vi "Stack_holderwise_total_bd_count_&_duration_Monthwise.vi"(0 "Refnum in":T1, 1 "BREAKDOWN_STK_HOLD_ID":i32=1, 2 "condition":string="Where BREAKDOWN_DATE between '%s'and '%s' and BREAKDOWN_STK_HOLD_ID ='%d'  ", 5 "Shift":string, 11 "error in (no error)":errorcluster) -> (4 "Refnum out":T1, 6 "Count out":string[](array[string]), 10 "appended array":dbl[](array[numeric]), 15 "error out":errorcluster)   [LabVIEW 2017]
uses:
  <vilib>/addons/database/Connection.llb/Conn ObjectReference.ctl
  <vilib>/addons/database/NI_Database_API.lvlib
panel:
  out "Table":string[][](array[string])
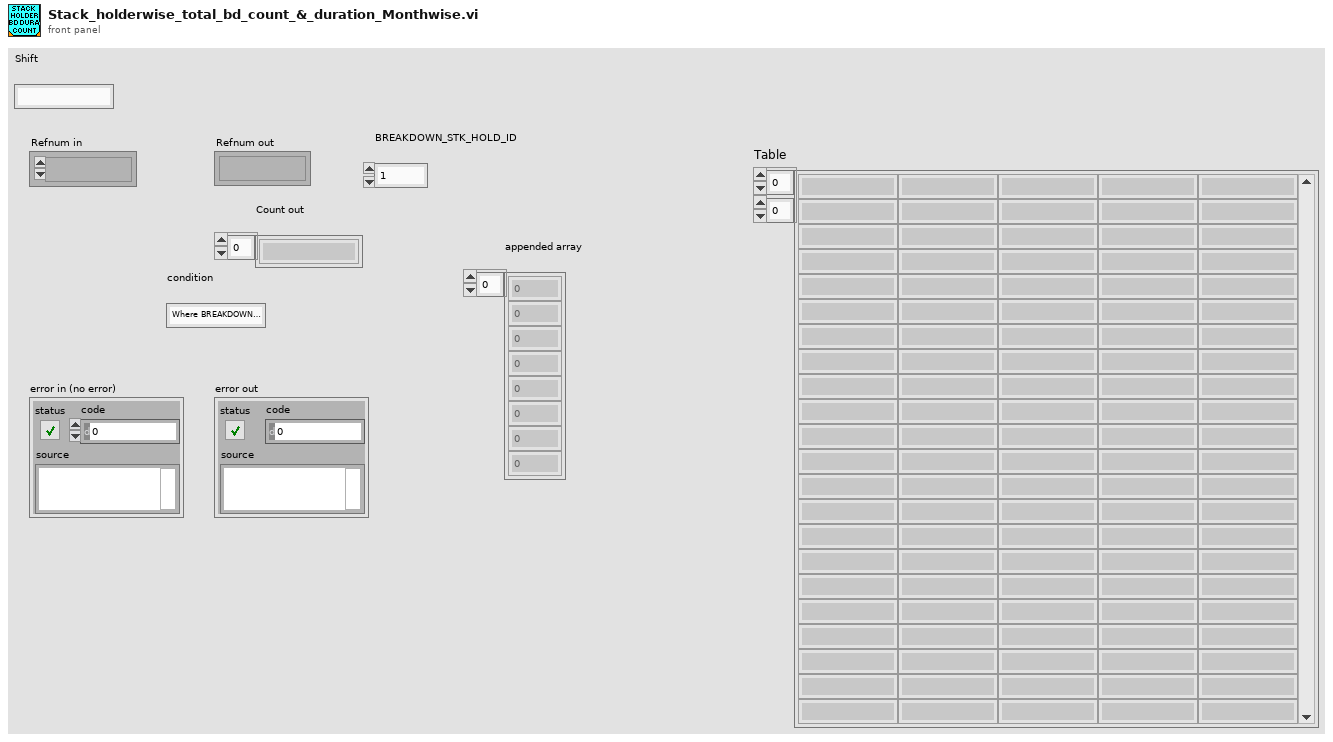
[diagram p1: front panel]
types:
  T1 = typedef "NI_Database_API.lvlib/Conn ObjectReference.ctl" = refnum<k1>
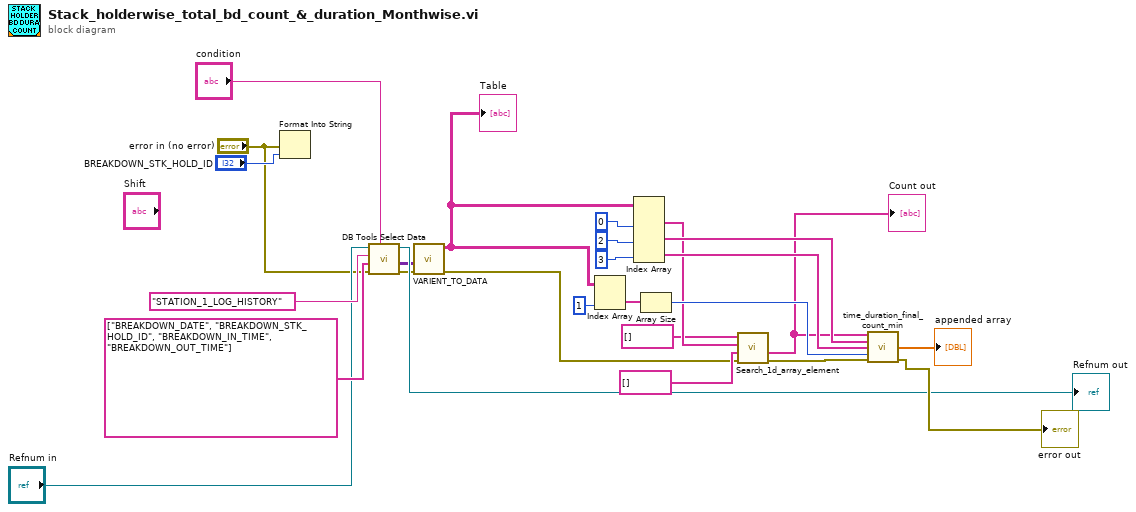
[diagram p0: block diagram]
diagram:
  n1 = Format Into String(error in="error in (no error)", "BREAKDOWN_STK_HOLD_ID") -> ()  [unwired: 2 in, 2 out]
  n2 = call <vilib>:"DB Tools Select Data.vi"("condition"="condition", "error in (no error)"="error in (no error)", "columns"=string[] ["BREAKDOWN_DATE", "BREAKDOWN_STK_HOLD_ID", "BREAKDOWN_IN_TIME", "BREAKDOWN_OUT_TIME"], "table"="STATION_1_LOG_HISTORY", "connection reference"="Refnum in") -> ("error out"=w6:errorcluster, "data"=w7:variant[][], "connection reference out"=→"Refnum out":T1)  [unwired: 1 in]
  n3 = call "VARIENT_TO_DATA.vi"("data"=w7, "error in (no error)"=w6) -> ("Table"=w23:string[][], "error out"=w24:errorcluster)  [unwired: 7 in]
  "Table" <- w23
  n4 = Index Array(array=w23, index (col)=1 ("disabled index (col)")) -> (element=w16:string[])  [unwired: 1 in]
  n5 = Index Array(array=w23, index (col) #1=0 ("disabled index (col)"), index (col) #2=2 ("disabled index (col)"), index (col) #3=3 ("disabled index (col)")) -> (element #1=w18:string[], element #2=w20:string[], element #3=w21:string[])  [unwired: 3 in]
  n6 = Array Size(array=w16) -> (size(s)=w22:i32)
  n7 = call "Search_1d_array_element.vi"("error in (no error)"=w24, "Count in"=string[] [] ("Count"), "BD Date"=w18, "Elements Found in"=string[] [] ("Elements Found")) -> ("error out"=w19:errorcluster, "Count out"=w5:string[])  [unwired: 3 in, 1 out]
  "Count out" <- w5
  n8 = call "time_duration_final_count_min.vi"("BD Count"=w5, "Intime"=w20, "OutTime"=w21, "bd array size"=w22, "error in (no error)"=w19) -> ("appended array"=→"appended array":dbl[], "error out"=→"error out":errorcluster)  [unwired: 7 in, 2 out]
